vi "ImagingTestSubVI.vi"() -> ()   [LabVIEW 2019]
uses:
  <vilib>/Utility/file.llb/Write Delimited Spreadsheet (I64).vi
  Program Files (x86)/National Instruments/LabVIEW 2019/ATMCD32D.dll
panel:
  in  "Tab Control":T1(tab)
  out "Expected position on spectrometer (pixels):":dbl
  in  "Harmonic":dbl min=10.0 max=40.0
  out "l (nm)":dbl
  out "E (J)":dbl
  out "E (eV)":dbl
  out "Nearest Harmonic of 800nm":dbl
  out "Cursor Position (pixels)":dbl
  out "Distance to nearest harmonic of 800nm (pixels)":dbl
  in  "Grating:":u16(ring) items=["Shimadzu 30-006  "]
  in  "Laser:":u16(ring) items=["800nm  "]
  in  "Trigger":u32(ring) items=["Internal", "External"]
  out "Initialize":u32
  in  "Exposure Time (secs)":sgl format="%.2f"
  out "Calculated Exposure Value":sgl format="%.5f"
  out "Get Acquired Data":u32
  out "Start Acquisition":u32
  out "Detector X Pixels":i32
  out "Check Timings":u32
  out "Set Acquisition Mode":u32
  out "Set Readout Mode":u32
  out "Set Trigger Mode":u32
  out "Set Exposure Time":u32
  out "Get Detector":u32
  out "Detector Y Pixels":i32
  out "Set Gate Mode":u32
  out "Set Image":u32
  out "Intensity Graph":i32[][](graph)
  out "Vertical Binned Waveform Graph":i32[](graph)
  out "Get Status":u32
  in  "Stop":bool
  in  "?":bool
  out "Camera Status:":bool
  out "Last Image Saved:":string
  out "Wavelength Graph":cluster{"No prefix":dbl, i32}[](graph)
  out "Energy Graph (eV)":cluster{"eV":dbl, i32}[](graph)
  out "Harmonics Graph":cluster{"No prefix":dbl, i32}[](graph)
  out "Status":u32
  # "Status"
  # "Return values"
  # "USB iStarIMAG32at.VI"
  # "Acquisition Mode: Single Scan\nReadout Mode: Full Resolution Image"
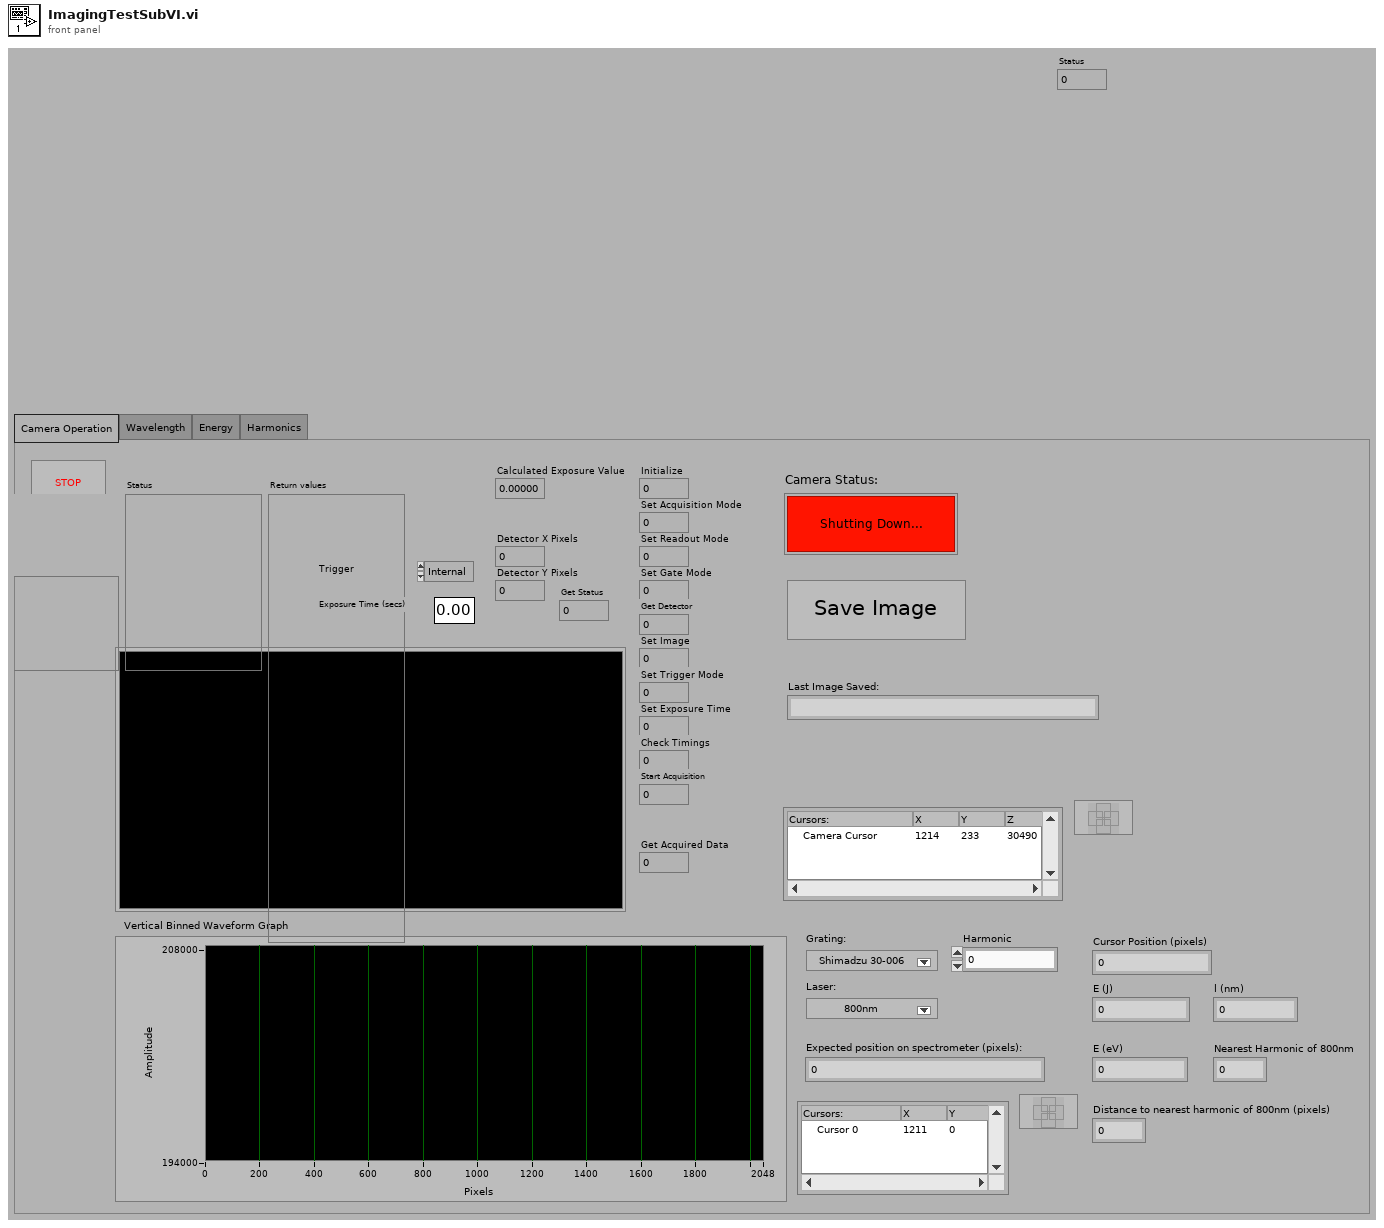
[diagram p1: front panel]
types:
  T1 = enum32{"Camera Operation", "Wavelength", "Energy", "Harmonics"}
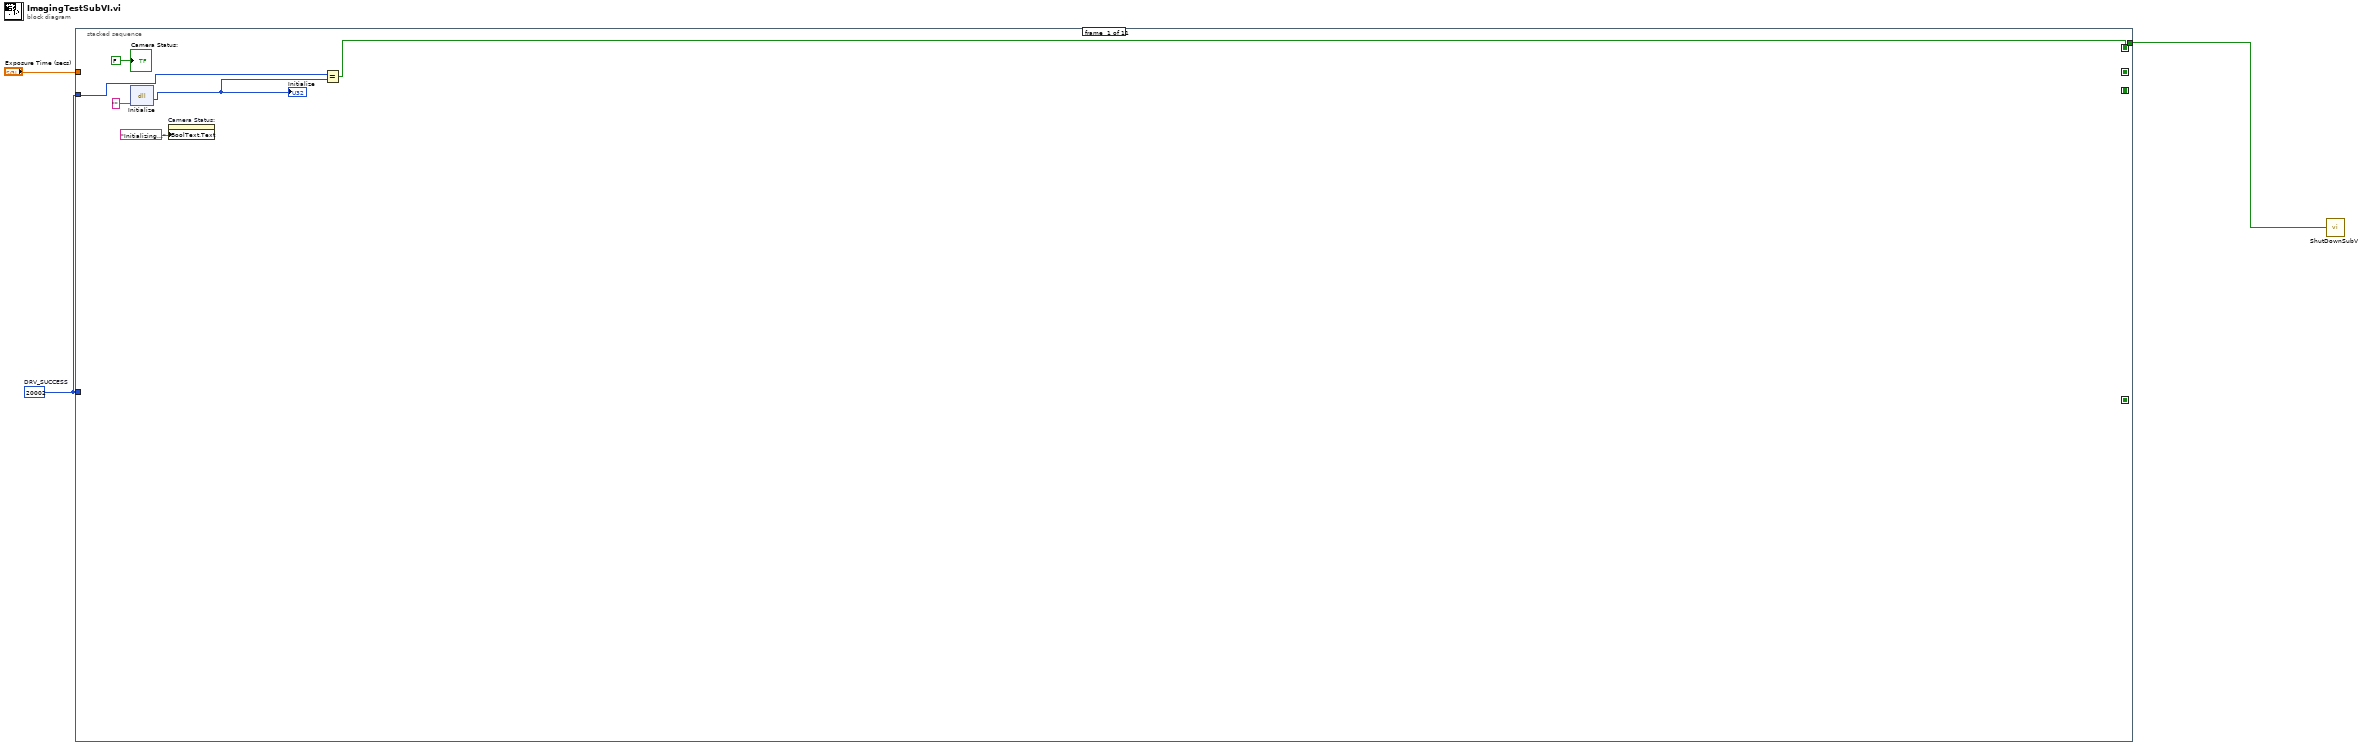
[diagram p0: block diagram]
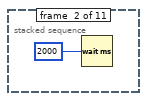
[diagram p2: hidden frame]
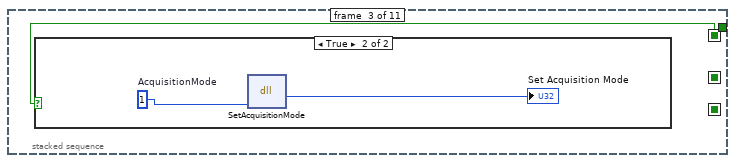
[diagram p3: hidden frame]
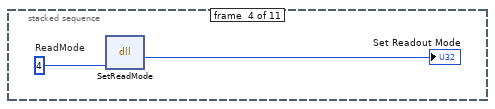
[diagram p5: hidden frame]
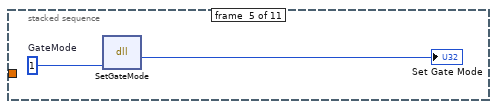
[diagram p6: hidden frame]
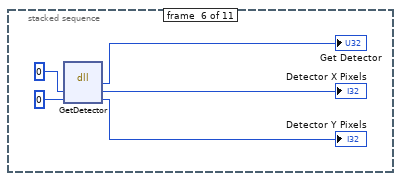
[diagram p7: hidden frame]
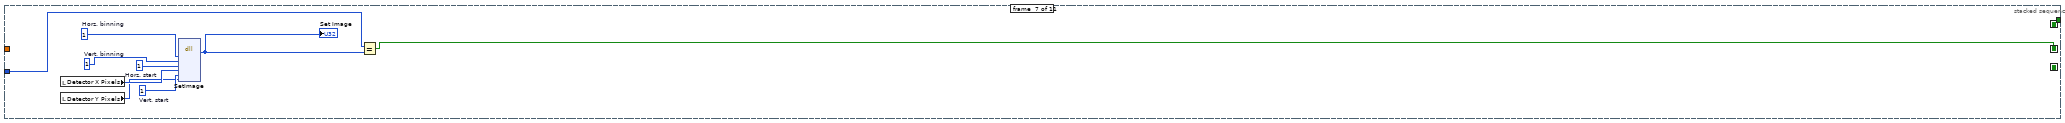
[diagram p8: hidden frame]
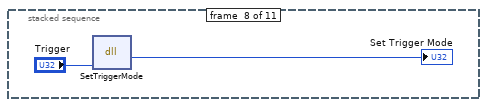
[diagram p9: hidden frame]
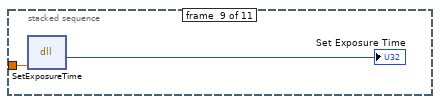
[diagram p10: hidden frame]
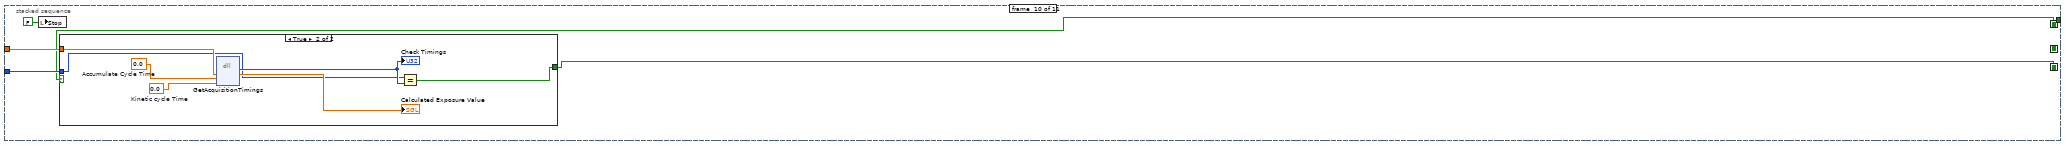
[diagram p11: hidden frame]
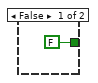
[diagram p12: hidden frame]
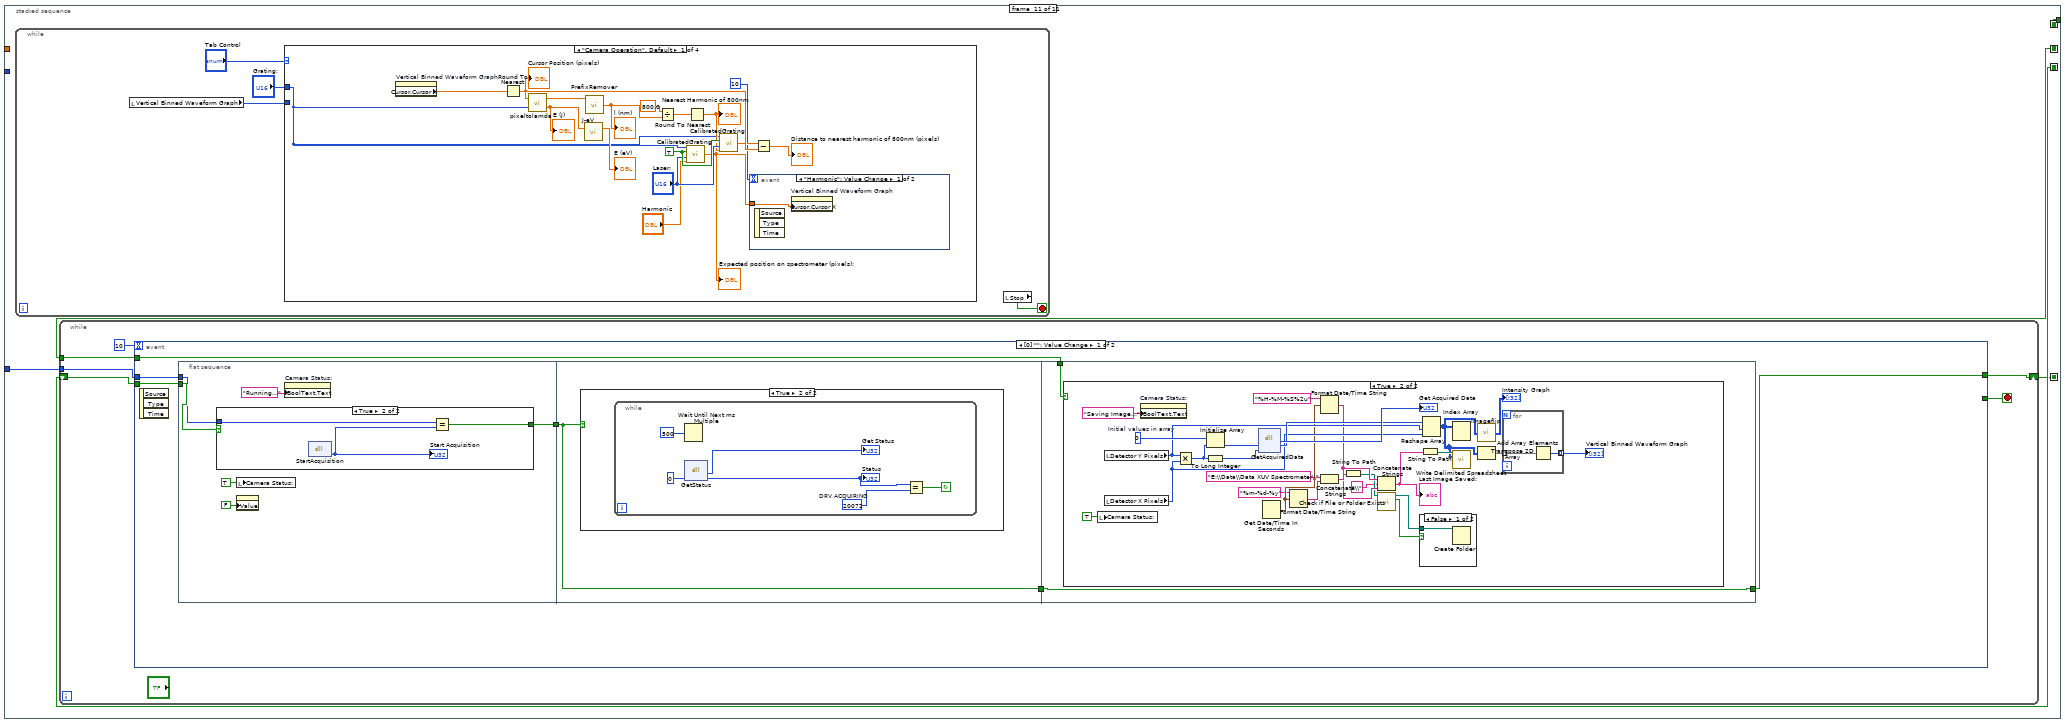
[diagram p13: hidden frame]
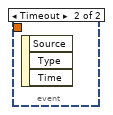
[diagram p14: hidden frame]
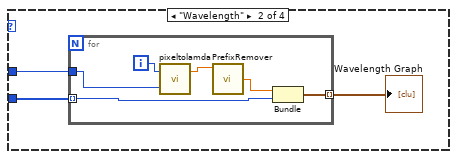
[diagram p15: hidden frame]
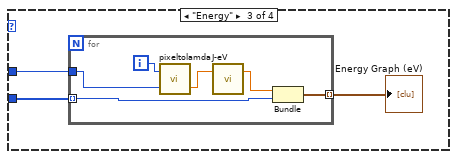
[diagram p16: hidden frame]
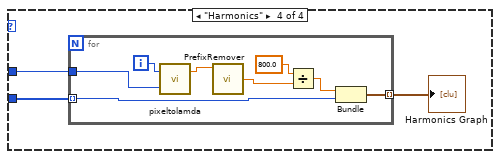
[diagram p17: hidden frame]
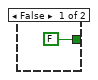
[diagram p18: hidden frame]
diagram:
  w2 = 20002  # DRV_SUCCESS
  n1 = stacked-sequence {
    seq-local: [w7 _ _ _ _ _ _ _ _ _ _] -> [_ _ w11 _ _ _ _ _ _ w37 w49]
    seq-local: [_ _ _ _ _ _ _ _ _ w38 _] -> [_ _ _ _ _ _ _ _ _ _ w53]
    seq-local: [_ _ _ _ _ _ _ _ _ _ w51] -> [_ _ _ _ _ _ _ _ _ _ _]
    seq-local: [_ _ _ _ _ _ w23 _ _ _ _] -> [_ _ _ _ _ _ _ _ _ _ w50]
    tunnel: "Exposure Time (secs)" -> [_ _ _ _ _ _ _ _ w35 w40 _]
    tunnel: w2 -> [w8 _ _ _ _ _ w25 _ _ w39 _]
    tunnel: w2 -> [_ _ _ _ _ _ _ _ _ _ w52]
    tunnel: [_ _ _ _ _ _ _ _ _ _ w49] -> w1
    frame #0 {
      n2 = dll-call lib="C:/Program Files (x86)/National Instruments/LabVIEW 2019/atmcd32d.dll" fn="Initialize" label="Call Library Function Initialize"("") -> (w9:u32)  [unwired: 4 in, 2 out]
      "Initialize" <- w9
      n3 = property on="Camera Status:" class="Bool (strict)"("BoolText.Text"="Initializing..." ("String")) -> ()  [unwired: 2 in, 2 out]
      n4 = Equal?(x=w8, y=w9) -> (x = y?=w7:bool)
      "Camera Status:" <- FALSE ("Camera Status:")
    }
    frame #1 {
      n5 = Wait (ms)(milliseconds to wait=u32 2000) -> ()  [unwired: 1 out]
    }
    frame #2 {
      n6 = case shown="True" w11 {
        frame False {
        }
        frame True {
          w13 = u16 1  # AcquisitionMode
          n7 = dll-call lib="C:/Program Files (x86)/National Instruments/LabVIEW 2019/atmcd32d.dll" fn="SetAcquisitionMode" label="Call Library Function SetAcquisitionMode"(w13) -> (→"Set Acquisition Mode":u32)  [unwired: 4 in, 2 out]
        }
      }
    }
    frame #3 {
      w15 = u16 4  # ReadMode
      n8 = dll-call lib="C:/Program Files (x86)/National Instruments/LabVIEW 2019/atmcd32d.dll" fn="SetReadMode" label="Call Library Function SetReadMode"(w15) -> (→"Set Readout Mode":u32)  [unwired: 4 in, 2 out]
    }
    frame #4 {
      w17 = u16 1  # GateMode
      n9 = dll-call lib="C:/Program Files (x86)/National Instruments/LabVIEW 2019/atmcd32d.dll" fn="SetGateMode" label="Call Library Function SetGateMode"(w17) -> (→"Set Gate Mode":u32)  [unwired: 4 in, 2 out]
    }
    frame #5 {
      n10 = dll-call lib="C:/Program Files (x86)/National Instruments/LabVIEW 2019/atmcd32d.dll" fn="GetDetector" label="Call Library FunctionGetDetector"(i16 0, i16 0) -> (→"Get Detector":u32, →"Detector X Pixels":i32, →"Detector Y Pixels":i32)  [unwired: 3 in, 2 out]
    }
    frame #6 {
      w28 = u16 1  # Vert. start
      w29 = u16 1  # Horz. start
      w30 = u16 1  # Vert. binning
      w31 = u16 1  # Horz. binning
      n11 = local read "Detector X Pixels"() -> (w27:i32)
      n12 = local read "Detector Y Pixels"() -> (w26:i32)
      n13 = dll-call lib="C:/Program Files (x86)/National Instruments/LabVIEW 2019/atmcd32d.dll" fn="SetImage" label="Call Library Function SetImage"(w31, w30, w29, w27, w28, w26) -> (w24:u32)  [unwired: 9 in, 2 out]
      "Set Image" <- w24
      n14 = Equal?(x=w25, y=w24) -> (x = y?=w23:bool)
    }
    frame #7 {
      n15 = dll-call lib="C:/Program Files (x86)/National Instruments/LabVIEW 2019/atmcd32d.dll" fn="SetTriggerMode" label="Call Library Function SetTrigger Mode"("Trigger") -> (→"Set Trigger Mode":u32)  [unwired: 4 in, 2 out]
    }
    frame #8 {
      n16 = dll-call lib="C:/Program Files (x86)/National Instruments/LabVIEW 2019/atmcd32d.dll" fn="SetExposureTime" label="Call Library FunctionSet Exposure Time"(w35) -> (→"Set Exposure Time":u32)  [unwired: 4 in, 2 out]
    }
    frame #9 {
      n17 = local write "Stop"(FALSE ("Stop")) -> ()
      n18 = case shown="True" w37 {
        tunnel: w40 -> [_ w45]
        tunnel: w39 -> [_ w42]
        tunnel: [FALSE w44] -> w38
        frame False {
        }
        frame True {
          w47 = sgl 0.0  # Accumulate Cycle Time
          w48 = sgl 0.0  # Kinetic cycle Time
          n19 = dll-call lib="C:/Program Files (x86)/National Instruments/LabVIEW 2019/atmcd32d.dll" fn="GetAcquisitionTimings" label="Call Library Function Check Timings"(w45, w47, w48) -> (w43:u32, →"Calculated Exposure Value":sgl)  [unwired: 5 in, 2 out]
          "Check Timings" <- w43
          n20 = Equal?(x=w42, y=w43) -> (x = y?=w44:bool)
        }
      }
    }
    frame #10 {
      n21 = while {
        stop <- w54 stop-if-true
        n22 = local read "Vertical Binned Waveform Graph"() -> (w56:i32[])
        n23 = case shown="\"Camera Operation\", Default" "Tab Control" {
          tunnel: w56 -> [_ w78 w87 w96]
          tunnel: "Grating:" -> [w58 w77 w86 w95]
          frame "Camera Operation", Default {
            w74 = TRUE
            n24 = property on="Vertical Binned Waveform Graph" class="WFGraph (strict)"() -> ("Cursor.Cursor X"=w71:dbl)  [unwired: 2 in, 2 out]
            n25 = Round To Nearest(number=w71) -> (nearest integer value=w64:dbl)
            "Cursor Position (pixels)" <- w64
            n26 = call "pixeltolamda.vi"("Grating:"=w58, "Pixel Postion"=w64) -> ("E (J)"=w66:dbl, "lamda (m)"=w72:dbl)
            "E (J)" <- w66
            n27 = call "J-eV.vi"("J"=w66) -> ("eV"=→"E (eV)":dbl)  [unwired: 1 in, 1 out]
            n28 = call "PrefixRemover.vi"("Nano"=w72) -> ("No prefix"=w67:dbl)  [unwired: 3 in]
            "l (nm)" <- w67
            n29 = Divide(x=800.0, y=w67) -> (x/y=w69:dbl)
            n30 = call "CalibratedGrating.vi"("Harmonic"="Harmonic", "Laser:"="Laser:", "Subvi?"=w74, "Grating:"=w58) -> ("Position on spectrometer (pixels):"=w60:dbl)
            "Expected position on spectrometer (pixels):" <- w60
            n31 = Round To Nearest(number=w69) -> (nearest integer value=w63:dbl)
            "Nearest Harmonic of 800nm" <- w63
            n32 = call "CalibratedGrating.vi"("Harmonic"=w63, "Laser:"="Laser:", "Subvi?"=w74, "Grating:"=w58) -> ("Position on spectrometer (pixels):"=w62:dbl)
            n33 = event shown="[0] \"Harmonic\": Value Change" {
              selector: _ -> [_ _]
              dyn-events: _ -> [_ _]
              timeout: 10 -> [_ _]
              tunnel: w60 -> [w75 _]
              event "Harmonic": Value Change {
                n34 = event-data() -> ()  [unwired: 1 in, 3 out]
                n35 = property on="Vertical Binned Waveform Graph" class="WFGraph (strict)"("Cursor.Cursor X"=w75) -> ()  [unwired: 2 in, 2 out]
              }
              event Timeout {
                n36 = event-data() -> ()  [unwired: 1 in, 3 out]
              }
            }
            n37 = Subtract(x=w62, y=w64) -> (x-y=→"Distance to nearest harmonic of 800nm (pixels)":dbl)
          }
          frame "Wavelength" {
            n38 = for {
              tunnel: w78 -> [w80] mode=indexing
              tunnel: w77 -> [w82]
              tunnel: [w79] -> w76 mode=indexing
              i -> [w81]
              n39 = call "pixeltolamda.vi"("Grating:"=w82, "Pixel Postion"=w81) -> ("lamda (m)"=w83:dbl)  [unwired: 1 out]
              n40 = call "PrefixRemover.vi"("Nano"=w83) -> ("No prefix"=w84:dbl)  [unwired: 3 in]
              n41 = Bundle("No prefix"=w84, w80) -> (w79:cluster{"No prefix":dbl, i32})  [unwired: 1 in]
            }
            "Wavelength Graph" <- w76
          }
          frame "Energy" {
            n42 = for {
              tunnel: w87 -> [w89] mode=indexing
              tunnel: w86 -> [w92]
              tunnel: [w88] -> w85 mode=indexing
              i -> [w93]
              n43 = call "pixeltolamda.vi"("Grating:"=w92, "Pixel Postion"=w93) -> ("E (J)"=w91:dbl)  [unwired: 1 out]
              n44 = call "J-eV.vi"("J"=w91) -> ("eV"=w90:dbl)  [unwired: 1 in, 1 out]
              n45 = Bundle("eV"=w90, w89) -> (w88:cluster{"eV":dbl, i32})  [unwired: 1 in]
            }
            "Energy Graph (eV)" <- w85
          }
          frame "Harmonics" {
            n46 = for {
              tunnel: w96 -> [w101] mode=indexing
              tunnel: w95 -> [w103]
              tunnel: [w100] -> w94 mode=indexing
              i -> [w102]
              n47 = call "pixeltolamda.vi"("Grating:"=w103, "Pixel Postion"=w102) -> ("lamda (m)"=w104:dbl)  [unwired: 1 out]
              n48 = call "PrefixRemover.vi"("Nano"=w104) -> ("No prefix"=w98:dbl)  [unwired: 3 in]
              n49 = Divide(x=800.0, y=w98) -> (x/y=w97:dbl)
              n50 = Bundle(w97, w101) -> (w100:cluster{dbl, i32})  [unwired: 1 in]
            }
            "Harmonics Graph" <- w94
          }
        }
        n51 = local read "Stop"() -> (w54:bool)
      }
      n52 = while {
        tunnel: w52 -> [w109]
        tunnel: w50 -> [w107]
        shift-right: [w108] -> w51
        shift-left: w53 -> [w110]
        stop <- w105 stop-if-true
        n53 = event shown="[0] \"\": Value Change" {
          selector: _ -> [_ _]
          dyn-events: _ -> [_ _]
          timeout: 10 -> [_ _]
          tunnel: w110 -> [w114 w171]
          tunnel: w109 -> [w113 w170]
          tunnel: [w112 w169] -> w108
          tunnel: w107 -> [w111 w168]
          tunnel: [_ w167] -> w105
          event Value Change {
            n54 = event-data() -> ()  [unwired: 1 in, 3 out]
            n55 = flat-sequence {
              tunnel: w114 -> [w122]
              tunnel: w113 -> [w121]
              tunnel: [w120] -> w116
              tunnel: w116 -> [w127]
              tunnel: [w127] -> w115
              tunnel: [w135] -> w112
              tunnel: w115 -> [w135]
              tunnel: w111 -> [w134]
              frame #0 {
                n56 = case shown="True" w122 {
                  tunnel: [FALSE w125] -> w120
                  tunnel: w121 -> [_ w124]
                  frame False {
                  }
                  frame True {
                    n57 = dll-call lib="C:/Program Files (x86)/National Instruments/LabVIEW 2019/atmcd32d.dll" fn="StartAcquisition" label="Call Library Function start acquisition"() -> (w126:u32)  [unwired: 3 in, 2 out]
                    "Start Acquisition" <- w126
                    n58 = Equal?(x=w124, y=w126) -> (x = y?=w125:bool)
                  }
                }
                n59 = local write "Camera Status:"(TRUE ("Camera Status:")) -> ()
                n60 = property class="Bool (strict)"("Value"=FALSE ("Take image")) -> ()  [unwired: 2 in, 2 out]
                n61 = property on="Camera Status:" class="Bool (strict)"("BoolText.Text"="Running..." ("Boolean Text.Text")) -> ()  [unwired: 2 in, 2 out]
              }
              frame #1 {
                n62 = case shown="True" w127 {
                  frame False {
                  }
                  frame True {
                    n63 = while {
                      stop <- w131 continue-if-true
                      w130 = u16 20072  # DRV ACQUIRING
                      n64 = Wait Until Next ms Multiple(millisecond multiple=u32 500) -> ()  [unwired: 1 out]
                      n65 = dll-call lib="C:/Program Files (x86)/National Instruments/LabVIEW 2019/atmcd32d.dll" fn="GetStatus" label="Call Library Function GetAcquisitionStatus"(u16 0) -> (→"Get Status":u32, w129:u32)  [unwired: 3 in, 2 out]
                      "Status" <- w129
                      n66 = Equal?(x=w129, y=w130) -> (x = y?=w131:bool)
                    }
                  }
                }
              }
              frame #2 {
                n67 = case shown="True" w134 {
                  frame False {
                  }
                  frame True {
                    w162 = 0  # Initial values in array
                    n68 = local write "Camera Status:"(TRUE ("Camera Status:")) -> ()
                    n69 = local read "Detector Y Pixels"() -> (w156:i32)
                    n70 = local read "Detector X Pixels"() -> (w155:i32)
                    n71 = property on="Camera Status:" class="Bool (strict)"("BoolText.Text"="Saving Image..." ("Boolean Text.Text")) -> ()  [unwired: 2 in, 2 out]
                    n72 = Multiply(x=w156, y=w155) -> (x*y=w158:i32)
                    n73 = To Long Integer(number=w158) -> (32bit integer=w159:i32)
                    n74 = Initialize Array "Initialize Array"(w162, w158) -> (w160:i32[])
                    n75 = dll-call lib="C:/Program Files (x86)/National Instruments/LabVIEW 2019/atmcd32d.dll" fn="GetAcquiredData" label="Call Library Function Get Acquired data"(w160, w159) -> (→"Get Acquired Data":u32, w157:i32[])  [unwired: 4 in, 2 out]
                    n76 = Get Date/Time In Seconds() -> (seconds since 1Jan1904=w152:timestamp)
                    n77 = Format Date/Time String(time format string (%c)="%m-%d-%y", seconds (now)=w152) -> (date/time string=w150:string)  [unwired: 1 in]
                    n78 = Format Date/Time String(time format string (%c)="%H-%M-%S%2u", seconds (now)=w152) -> (date/time string=w151:string)  [unwired: 1 in]
                    n79 = Concatenate Strings("E:\\Data\\Data XUV Spectrometer\\" ("string"), w150) -> (w153:string)
                    n80 = String To Path(string=w153) -> (path=w149:path)
                    n81 = Concatenate Strings(w153, "\\" ("string"), w151) -> (w154:string)
                    "Last Image Saved:" <- w154
                    n82 = call <vilib>:"Check if File or Folder Exists.vi"("path"=w149) -> ("file or folder exists?"=w147:bool, "dup path"=w148:path)  [unwired: 8 in, 1 out]
                    n83 = case shown="False" w147 {
                      tunnel: w148 -> [w165 _]
                      frame False {
                        n84 = Create Folder(path (use dialog)=w165) -> ()  [unwired: 2 in, 3 out]
                      }
                      frame True {
                      }
                    }
                    n85 = String To Path(string=w154) -> (path=w142:path)
                    n86 = Reshape Array(w157, w156, w155) -> (w137:i32[][])
                    n87 = Index Array(array=w137) -> ()  [unwired: 2 in, 1 out]
                    n88 = call-poly <vilib>:"Write Delimited Spreadsheet.vi"("file path (dialog if empty)"=w142, "2D data"=w137) -> ()  [unwired: 12 in, 2 out]
                    n89 = call "Imageflip.vi"("2D array"=w137) -> ("transposed array"=→"Intensity Graph":i32[][])
                    n90 = Transpose 2D Array(2D array=w137) -> (transposed array=w141:i32[][])
                    n91 = for {
                      tunnel: w141 -> [w164] mode=indexing
                      tunnel: [w163] -> w140 mode=indexing
                      n92 = Add Array Elements(numeric array=w164) -> (sum=w163:i32)
                    }
                    "Vertical Binned Waveform Graph" <- w140
                  }
                }
              }
            }
          }
          event Timeout {
            n93 = event-data() -> ()  [unwired: 1 in, 3 out]
            n94 = flat-sequence {
              tunnel: w171 -> [w178]
              tunnel: w170 -> [w177]
              tunnel: [w176] -> w173
              tunnel: w173 -> [w183]
              tunnel: [w183] -> w172
              tunnel: w172 -> [w190]
              tunnel: w168 -> [w191]
              tunnel: [w190] -> w166
              tunnel: ["Stop"] -> w167
              tunnel: [w216] -> w169
              tunnel: w166 -> [w216]
              frame #0 {
                n95 = case shown="True" w178 {
                  tunnel: [FALSE w182] -> w176
                  tunnel: w177 -> [_ w181]
                  frame False {
                  }
                  frame True {
                    n96 = dll-call lib="C:/Program Files (x86)/National Instruments/LabVIEW 2019/atmcd32d.dll" fn="StartAcquisition" label="Call Library Function start acquisition"() -> (w180:u32)  [unwired: 3 in, 2 out]
                    n97 = local write "Start Acquisition"(w180) -> ()
                    n98 = Equal?(x=w181, y=w180) -> (x = y?=w182:bool)
                  }
                }
                n99 = local write "Camera Status:"(TRUE ("Camera Status:")) -> ()
                n100 = property on="Camera Status:" class="Bool (strict)"("BoolText.Text"="Running..." ("Boolean Text.Text")) -> ()  [unwired: 2 in, 2 out]
              }
              frame #1 {
                n101 = case shown="True" w183 {
                  frame False {
                  }
                  frame True {
                    n102 = while {
                      stop <- w187 continue-if-true
                      w186 = u16 20072  # DRV ACQUIRING
                      n103 = Wait Until Next ms Multiple(millisecond multiple=u32 500) -> ()  [unwired: 1 out]
                      n104 = dll-call lib="C:/Program Files (x86)/National Instruments/LabVIEW 2019/atmcd32d.dll" fn="GetStatus" label="Call Library Function GetAcquisitionStatus"(u16 0) -> (w185:u32, w184:u32)  [unwired: 3 in, 2 out]
                      n105 = local write "Status"(w184) -> ()
                      n106 = local write "Get Status"(w185) -> ()
                      n107 = Equal?(x=w184, y=w186) -> (x = y?=w187:bool)
                    }
                  }
                }
              }
              frame #2 {
                n108 = case shown="True" w191 {
                  frame False {
                  }
                  frame True {
                    w206 = 0  # Initial values in array
                    n109 = local read "Detector Y Pixels"() -> (w201:i32)
                    n110 = local read "Detector X Pixels"() -> (w200:i32)
                    n111 = Multiply(x=w201, y=w200) -> (x*y=w203:i32)
                    n112 = Initialize Array "Initialize Array"(w206, w203) -> (w205:i32[])
                    n113 = To Long Integer(number=w203) -> (32bit integer=w204:i32)
                    n114 = dll-call lib="C:/Program Files (x86)/National Instruments/LabVIEW 2019/atmcd32d.dll" fn="GetAcquiredData" label="Call Library Function Get Acquired data"(w205, w204) -> (w198:u32, w202:i32[])  [unwired: 4 in, 2 out]
                    n115 = local write "Get Acquired Data"(w198) -> ()
                    n116 = Reshape Array(w202, w201, w200) -> (w192:i32[][])
                    n117 = Index Array(array=w192) -> ()  [unwired: 2 in, 1 out]
                    n118 = Array Max & Min(array=w192) -> (max value=w196:i32)  [unwired: 3 out]
                    n119 = Transpose 2D Array(2D array=w192) -> (transposed array=w199:i32[][])
                    n120 = call "Imageflip.vi"("2D array"=w192) -> ("transposed array"=w193:i32[][])
                    n121 = for {
                      tunnel: w199 -> [w214] mode=indexing
                      tunnel: [w213] -> w197 mode=indexing
                      n122 = Add Array Elements(numeric array=w214) -> (sum=w213:i32)
                    }
                    n123 = local write "Intensity Graph"(w193) -> ()
                    n124 = Greater?(x=w196, y=64900) -> (0:w194:bool)
                    n125 = case shown="True" w194 {
                      frame False {
                      }
                      frame True {
                        n126 = local write "Camera Status:"(FALSE ("Camera Status:")) -> ()
                        n127 = property on="Camera Status:" class="Bool (strict)"("BoolText.Text"="Saturated!" ("Boolean Text.Text")) -> ()  [unwired: 2 in, 2 out]
                        n128 = Two Button Dialog(message="Camera is saturating! Reduce photon flux!", 1:"I've fixed it, and I want to continue" ("message"), 2:"Shut Down Camera" ("T button name (\"OK\")")) -> (T button?=w208:bool)
                        n129 = local write "Stop"(w208) -> ()
                      }
                    }
                    n130 = local write "Vertical Binned Waveform Graph"(w197) -> ()
                  }
                }
              }
              frame #3 {
              }
            }
          }
        }
      }
    }
  }
  n131 = call "ShutDownSubVI.vi"("Initialize (bool 1)"=w1) -> ()  [unwired: 2 in]
